vi "FetchVal34980.vi"(2 "error in (no error)":errorcluster, 3 "Circuit ID":i32=1016 format="%_4g") -> (0 "Error out":errorcluster, 1 "Value":dbl format="%#_10e")   [LabVIEW 2009]
doc: "Reads a value from the 34980. \nAssumes that you have scanned the 34980 to store the values."
panel:
  # "This assumes you have already scanned the 34980"
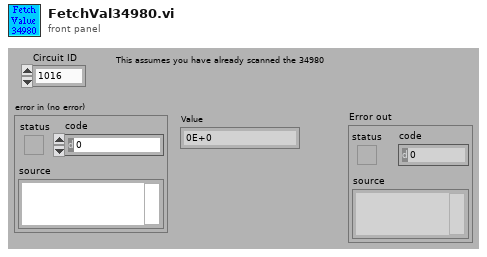
[diagram p1: front panel]
types:
  T1 = enum16{"N1911A", "Siggen", "34980a", "E4418B", "Rvp8"}
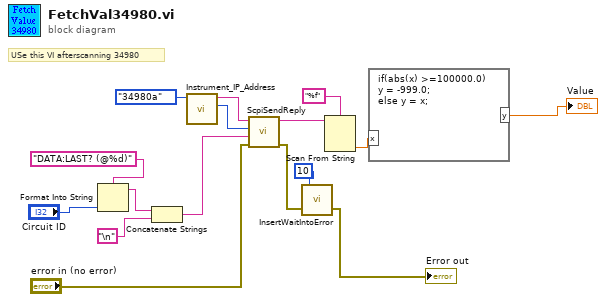
[diagram p0: block diagram]
diagram:
  # "USe this VI afterscanning 34980"
  n1 = Format Into String(format string="DATA:LAST? (@%d)", "Circuit ID") -> (resulting string=w11:string)  [unwired: 2 in, 1 out]
  n2 = Concatenate Strings(w11, "\n") -> (w9:string)
  n3 = call "Instrument_IP_Address.vi"("Instrument"=T1."34980a") -> ("Port"=w1:u16, "IP Address"=w2:string)  [unwired: 9 in]
  n4 = call "ScpiSendReply.vi"("error in (no error)"="error in (no error)", "Command"=w9, "TCP port"=w1, "IP Address"=w2) -> ("Error out"=w8:errorcluster, "Reply"=w15:string)  [unwired: 5 in]
  n5 = call "InsertWaitIntoError.vi"("error in (no error)"=w8, "Wait (msecs)"=10) -> ("error out"=→"Error out":errorcluster)  [unwired: 1 in]
  n6 = Scan From String(format string="%f", input string=w15) -> (output 1=w5:dbl)  [unwired: 3 in, 3 out]
  n7 = formula code="if(abs(x) >=100000.0)\ny = -999.0;\nelse y = x;"("x"=w5) -> ("y"=→"Value":dbl)
